vi "Enqueue.vi"(8 "Error In":errorcluster, 10 "Data":variant, 11 "Command":T1) -> (0 "Error Out":errorcluster)   [LabVIEW 2023, in "Error Manager.lvlib" / "Error Window Loop Queue.lvclass"]
doc: "Issues a command by enqueuing into the module's command queue. The command should be received by calling the 'Dequeue' VI."
uses:
  Error Window Loop Queue.lvclass
  Command (enum).ctl
  Message (cluster).ctl
  Queue Reference (library variable).vi
  Error Window Loop Queue.lvclass/Error Window Loop Queue.ctl
panel:
  # "Input\nInputs to the VI"
  # "Development\nControls or indicators that are useful for development or testing, but which are not outputs of the VI."
  # "Output\nOutputs of the VI"
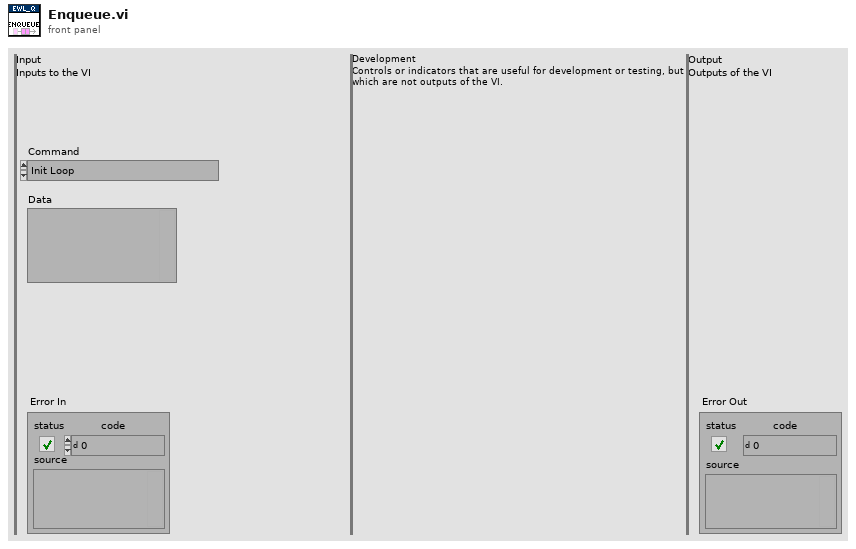
[diagram p1: front panel]
types:
  T1 = typedef "Error Manager.lvlib/Error Window Loop Queue.lvclass/Command (enum).ctl" = enum16{"Init Loop", "Close Loop", "Show Error Window"}
  T2 = typedef "Error Manager.lvlib/Error Window Loop Queue.lvclass/Message (cluster).ctl" = cluster{"Command":T1, "Data":variant}
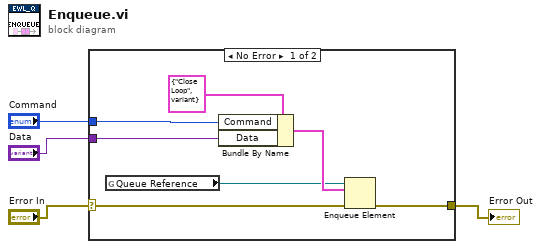
[diagram p0: block diagram]
diagram:
  n1 = case shown="No Error" "Error In" {
    selector: "Error In" -> [w11 w12]
    tunnel: [w10 w12] -> w3
    tunnel: "Command" -> [w7 _]
    tunnel: "Data" -> [w6 _]
    frame No Error {
      n2 = global read "Queue Reference (library variable).vi" "Queue Reference"() -> (w5:refnum<queue>)
      n3 = Bundle By Name(cluster=T2 {"Command"=enum."Close Loop", "Data"=variant} ("Queue Message"), "Command"=w7, "Data"=w6) -> (w8:T2)
      n4 = Enqueue Element(queue=w5, element=w8, error in (no error)=w11) -> (error out=w10:errorcluster)  [unwired: 1 in, 2 out]
    }
    frame Error {
    }
  }
  "Error Out" <- w3
